vi "Clusters to JSON Objects or Arrays.vi"() -> ()   [LabVIEW 2017]
doc: "Shows how LabVIEW Clusters can be saved as either JSON Objects or Arrays, depending on if cluster elements have names."
uses:
  7b028778-7c9b-4972-88c4-ca80fa94cd03.vi
  289da8a0-1b3f-4f96-b1eb-aa7cb4e9c5df.vi
  088bd8c3-5f0a-4b13-bcc9-44c75584851b.vi
  bbd2c762-b014-436a-9365-5811203f0396.vi
  Variant to JSON Text.vi
  JSON text to Variant.vi
panel:
  out "Cluster of unnamed elements":cluster{string, dbl, string}
  out "Object Data":T1
  out "<JSON> Array":string
  out "<JSON> Object":string
  # "Run this VI, then see block diagram:"
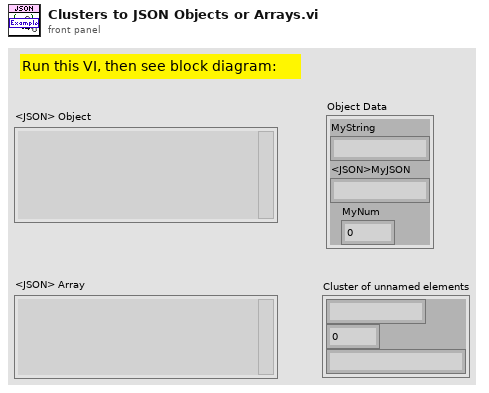
[diagram p1: front panel]
types:
  T1 = cluster{"MyString":string, "<JSON>MyJSON":string, "MyNum":dbl}
  T2 = cluster{"MyString":string, "MyNum":dbl, "<JSON>MyJSON":string}
  T3 = cluster{string, "MyNum":dbl, "<JSON>MyJSON":string}
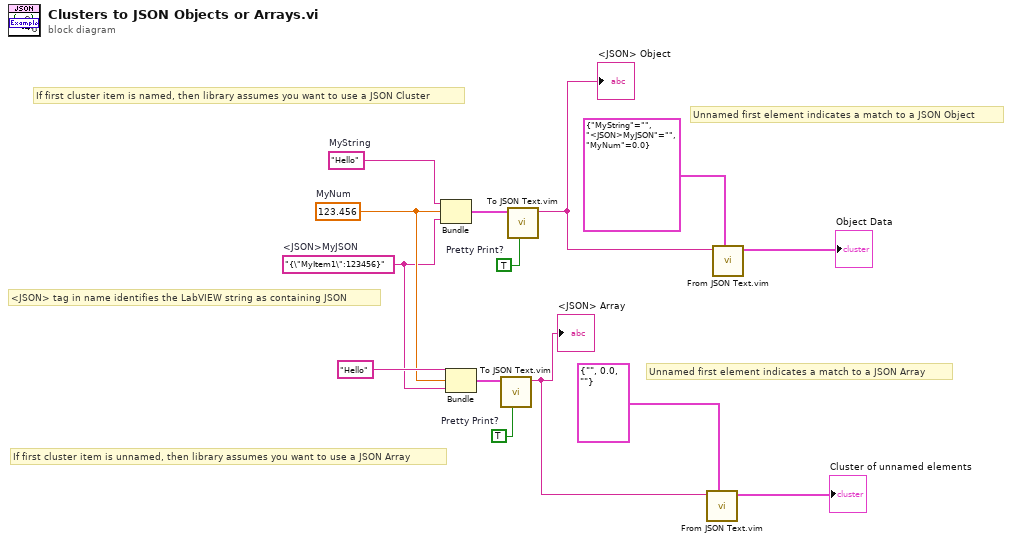
[diagram p0: block diagram]
diagram:
  w1 = TRUE  # Pretty Print?
  w2 = TRUE  # Pretty Print?
  w11 = "{\"MyItem1\":123456}"  # <JSON>MyJSON
  w12 = 123.456  # MyNum
  w14 = "Hello"  # MyString
  # "Unnamed first element indicates a match to a JSON Object"
  # "If first cluster item is named, then library assumes you want to use a JSON Cluster"
  # "Unnamed first element indicates a match to a JSON Array"
  # "<JSON> tag in name identifies the LabVIEW string as containing JSON"
  # "If first cluster item is unnamed, then library assumes you want to use a JSON Array"
  n1 = Bundle("MyString"=w14, "MyNum"=w12, "<JSON>MyJSON"=w11) -> (w5:T2)  [unwired: 1 in]
  n2 = Bundle("Hello", "MyNum"=w12, "<JSON>MyJSON"=w11) -> (w10:T3)  [unwired: 1 in]
  n3 = call "To JSON Text.vim"("Pretty Print?"=w1, "Anything"=w10) -> ("<JSON>"=w6:string)  [unwired: 8 in, 1 out]
  "<JSON> Array" <- w6
  n4 = call "To JSON Text.vim"("Pretty Print?"=w2, "Anything"=w5) -> ("<JSON>"=w7:string)  [unwired: 8 in, 1 out]
  "<JSON> Object" <- w7
  n5 = call "From JSON Text.vim"("Data Type and Default Value"=cluster{string, dbl, "<JSON>":string} {"", 0.0, "<JSON>"=""} ("output cluster"), "JSON"=w6) -> ("Data out"=→"Cluster of unnamed elements":cluster{string, dbl, "<JSON>":string})  [unwired: 8 in, 1 out]
  n6 = call "From JSON Text.vim"("Data Type and Default Value"=T1 {"MyString"="", "<JSON>MyJSON"="", "MyNum"=0.0} ("output cluster"), "JSON"=w7) -> ("Data out"=→"Object Data":T1)  [unwired: 8 in, 1 out]
